vi "sendValue.vi"(8 "error in (no error)":errorcluster, 10 "data":variant, 11 "emergencyStop in":refnum<class "emergencyStop.lvclass">) -> (0 "error out":errorcluster, 2 "function return":i32, 3 "emergencyStop out":refnum<class "emergencyStop.lvclass">)   [LabVIEW 2016, in "SALLV_AtDome_Messaging.lvlib" / "emergencyStop.lvclass"]
uses:
  emergencyStop.lvclass
  ts_sallv_AtDome/DataTypes/logevent_emergencyStop.ctl
  ts_sallv_AtDome/SALLV_AtDome.lvlib
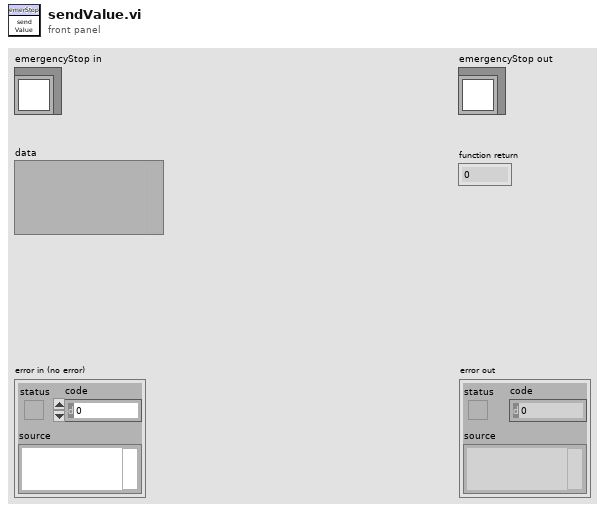
[diagram p1: front panel]
types:
  T1 = typedef "SALLV_AtDome.lvlib/logevent_emergencyStop.ctl" = cluster{"active":bool, "priority":i32}
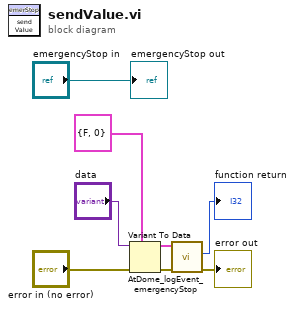
[diagram p0: block diagram]
diagram:
  n1 = Variant To Data(error in="error in (no error)", type=T1 {"active"=FALSE, "priority"=0} ("logevent_emergencyStop_Ctl"), Variant="data") -> (data=w2:T1, error out=w5:errorcluster)
  n2 = call "AtDome_logEvent_emergencyStop.vi"("error in (no error)"=w5, "logevent_emergencyStop_Ctl"=w2) -> ("error out"=→"error out":errorcluster, "function return"=→"function return":i32)  [unwired: 7 in, 1 out]
  "emergencyStop out" <- "emergencyStop in"
